vi "ACT_Loop.vi"() -> ()   [LabVIEW 2023, in "Grabber_ACT.lvlib"]
uses:
  Grabber_ACT.lvlib
  Cluster_CMD_ACT_Data.ctl
  Shared Code/TypeDefs/ENUM_Grabber_CMD_Mode Select.ctl
  Shared Code/TypeDefs/Cluster_Grabber_Config FX Values.ctl
  Shared Code/TypeDefs/Cluser_CAN Data.ctl
  Shared Code/TypeDefs/Cluster_Config Motor Output.ctl
  <vilib>/Rock Robotics/WPI/ThirdParty/Phoenix-LabVIEW/Motor Controller/Controls/CTRE_Phoenix_MotorControl_TalonFXInvertType.ctl
  <vilib>/Rock Robotics/WPI/ThirdParty/Phoenix-LabVIEW/Motor Controller/Controls/CTRE_Phoenix_MotorControl_NeutralMode.ctl
  Shared Code/TypeDefs/Cluster_FWD  REV Values.ctl
  Shared Code/TypeDefs/Cluser_FX Config_Current Limits.ctl
  Shared Code/TypeDefs/Cluster_Grabber HW Outputs.ctl
  Shared Code/TypeDefs/Cluster_FX Sensor Values.ctl
  Shared Code/TypeDefs/Cluster_FX CloseLoop Values.ctl
  Shared Code/TypeDefs/Cluster_FX Current Values.ctl
  Shared Code/TypeDefs/Cluster_Grabber_SW Outputs.ctl
  Shared Code/TypeDefs/Cluster_Grabber_Config SW Values.ctl
  ENUM_ACT_State.ctl
  <vilib>/Rock Robotics/WPI/MotorControl/WPI_MotorControlDeviceRef.ctl
  <vilib>/Rock Robotics/WPI/MotorControl/WPI_MotorControlType.ctl
  <vilib>/Rock Robotics/SystemInterfaces/DIO/FPGA_DIOPWMChannel.ctl
  <vilib>/Rock Robotics/WPI/PWM/WPI_PWMDeadband.ctl
  <vilib>/Rock Robotics/SystemInterfaces/DIO/FPGA_DIOChannel.ctl
  <vilib>/Rock Robotics/WPI/ThirdParty/Phoenix-LabVIEW/Motor Controller/Controls/CTRE_Phoenix_MotorControl_ControlMode.ctl
  ENUM_ACT_Action.ctl
  e7fa0f6b-fe57-4250-9995-b404d65a8362.vi
  4f1f8321-3dc8-4b28-8619-20673fc77ec2.vi
  6201c2b1-dcd8-4430-86f1-9b4ee56c7753.vi
  b5508d6c-c1cc-4273-80c5-2077d34e1483.vi
  36677ea0-a1a5-47a3-bc56-4475cb7c281e.vi
  5f725c2a-0ce1-4524-8967-e83b15fdce90.vi
  573e44c0-11f4-4bd9-ad56-904ec25dba75.vi
  e7494af9-f670-4352-9dfa-ae6ce50709ea.vi
  <vilib>/Utility/error.llb/Trim Whitespace.vi
  36677ea0-a1a5-47a3-bc56-4475cb7c281e.vi/958b2683-dd4b-41b7-8ed1-41c95f63cef0.vi
  36677ea0-a1a5-47a3-bc56-4475cb7c281e.vi/95f5fa9b-6175-4b34-88ee-cece92c38279.vi
  5f725c2a-0ce1-4524-8967-e83b15fdce90.vi/958b2683-dd4b-41b7-8ed1-41c95f63cef0.vi
  5f725c2a-0ce1-4524-8967-e83b15fdce90.vi/95f5fa9b-6175-4b34-88ee-cece92c38279.vi
  573e44c0-11f4-4bd9-ad56-904ec25dba75.vi/958b2683-dd4b-41b7-8ed1-41c95f63cef0.vi
  573e44c0-11f4-4bd9-ad56-904ec25dba75.vi/95f5fa9b-6175-4b34-88ee-cece92c38279.vi
  e7494af9-f670-4352-9dfa-ae6ce50709ea.vi/958b2683-dd4b-41b7-8ed1-41c95f63cef0.vi
  e7494af9-f670-4352-9dfa-ae6ce50709ea.vi/95f5fa9b-6175-4b34-88ee-cece92c38279.vi
  <vilib>/Utility/error.llb/Trim Whitespace One-Sided.vi
  36677ea0-a1a5-47a3-bc56-4475cb7c281e.vi/95f5fa9b-6175-4b34-88ee-cece92c38279.vi/1c6bd52c-bbca-4d4a-a290-93ea2703fded.vi
  36677ea0-a1a5-47a3-bc56-4475cb7c281e.vi/95f5fa9b-6175-4b34-88ee-cece92c38279.vi/47c2b0d5-b5fa-444e-9535-611565d375db.vi
  5f725c2a-0ce1-4524-8967-e83b15fdce90.vi/95f5fa9b-6175-4b34-88ee-cece92c38279.vi/1c6bd52c-bbca-4d4a-a290-93ea2703fded.vi
  5f725c2a-0ce1-4524-8967-e83b15fdce90.vi/95f5fa9b-6175-4b34-88ee-cece92c38279.vi/47c2b0d5-b5fa-444e-9535-611565d375db.vi
  573e44c0-11f4-4bd9-ad56-904ec25dba75.vi/95f5fa9b-6175-4b34-88ee-cece92c38279.vi/1c6bd52c-bbca-4d4a-a290-93ea2703fded.vi
  573e44c0-11f4-4bd9-ad56-904ec25dba75.vi/95f5fa9b-6175-4b34-88ee-cece92c38279.vi/47c2b0d5-b5fa-444e-9535-611565d375db.vi
  e7494af9-f670-4352-9dfa-ae6ce50709ea.vi/95f5fa9b-6175-4b34-88ee-cece92c38279.vi/1c6bd52c-bbca-4d4a-a290-93ea2703fded.vi
  e7494af9-f670-4352-9dfa-ae6ce50709ea.vi/95f5fa9b-6175-4b34-88ee-cece92c38279.vi/47c2b0d5-b5fa-444e-9535-611565d375db.vi
  RoboRIO Utilities/Global_STOP.vi
  Global_CMD_ACT_Data In.vi
  <vilib>/Utility/Data Type/Get Type Information.vi
  Shared Code/Utility/RWA/RWA/File/RWA_PC FIle Read String.vi
  Shared Code/Utility/RWA/RWA/Read Write Anything/RWA_File String.vi
  Shared Code/Utility/RWA/RWA/File/RWA_PC File Write String.vi
  Global_ACT_Data Out.vi
  <vilib>/Comparison/Equal/Equal Functor/Equal Functor.lvclass
panel:
  in  "Positon GO":bool
  in  "CMD Override":enum32{"None", "Intake", "Eject", "STOP"}(tab)
  out "Current Time":timestamp
  in  "SW Config":T1={"GrabberSW Ver"=230304152401, "Intake Speed"=0.4, "Eject Speed"=0.1, "Current Limit Velocity"=-12000, "Current Limit"=4.0, "Current Starting"=40.0, "Max Full Time(S)"=0.5}
  out "SW Output":T2
  out "Sensor Read time":dbl format="%.3g"
  out "HW Outputs":T3
  in  "Read Saved Config":bool
  in  "Update Config":bool
  in  "HW Config":T7 {"Output"."Min"."REV" format="%.2f"; "Output"."Min"."FWD" format="%.2f"; "Output"."Max"."REV" format="%.2f"; "Output"."Max"."FWD" format="%.2f"}
  out "CMD":T14
  out "Cycle Time (S)":dbl format="%.3g"
  # "Intake"
  # "Eject"
  # "STOP"
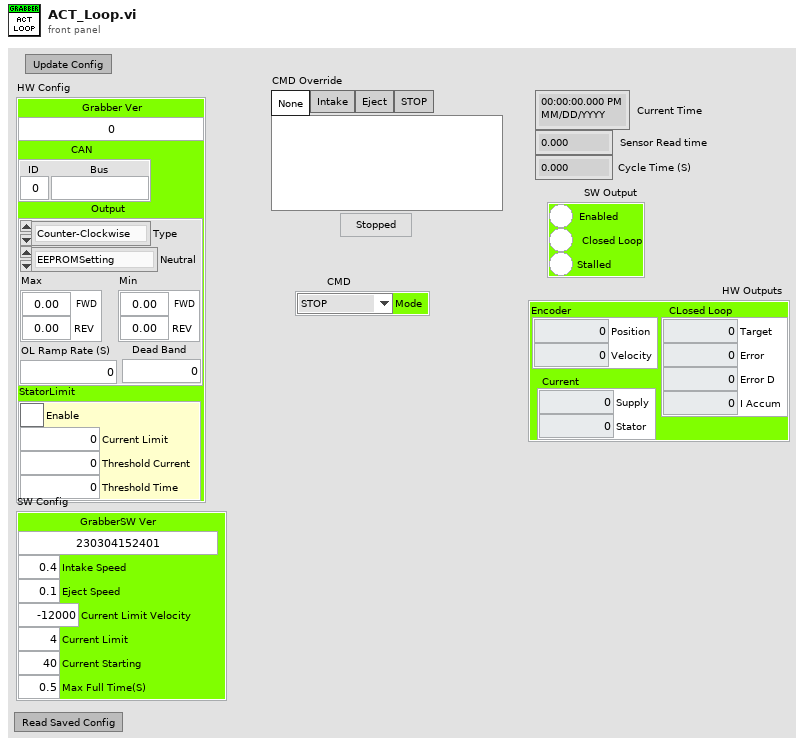
[diagram p1: front panel]
types:
  T1 = typedef "Cluster_Grabber_Config SW Values.ctl" = cluster{"GrabberSW Ver":u64, "Intake Speed":dbl, "Eject Speed":dbl, "Current Limit Velocity":i32, "Current Limit":dbl, "Current Starting":dbl, "Max Full Time(S)":dbl}
  T2 = typedef "Cluster_Grabber_SW Outputs.ctl" = cluster{"Enabled":bool, "Closed Loop":bool, "Stalled":bool}
  T3 = typedef "Cluster_Grabber HW Outputs.ctl" = cluster{"Encoder":T4, "CLosed Loop":T5, "Current":T6}
  T4 = typedef "Cluster_FX Sensor Values.ctl" = cluster{"Position":i32, "Velocity":i32}
  T5 = typedef "Cluster_FX CloseLoop Values.ctl" = cluster{"Target":dbl, "Error":i32, "Error D":dbl, "I Accum":dbl}
  T6 = typedef "Cluster_FX Current Values.ctl" = cluster{"Supply":dbl, "Stator":dbl}
  T7 = typedef "Cluster_Grabber_Config FX Values.ctl" = cluster{"Grabber Ver":u64, "CAN":T8, "Output":T9, "StatorLimit":T13}
  T8 = typedef "Cluser_CAN Data.ctl" = cluster{"ID":u8, "Bus":string}
  T9 = typedef "Cluster_Config Motor Output.ctl" = cluster{"Type":T10, "Neutral":T11, "Max":T12, "Min":T12, "OL Ramp Rate (S)":dbl, "Dead Band":dbl}
  T10 = typedef "CTRE_Phoenix_MotorControl_TalonFXInvertType.ctl" = enum16{"Counter-Clockwise", "Clockwise"}
  T11 = typedef "CTRE_Phoenix_MotorControl_NeutralMode.ctl" = enum8{"EEPROMSetting", "Override to Coast", "Override to Brake"}
  T12 = typedef "Cluster_FWD  REV Values.ctl" = cluster{"FWD":dbl, "REV":dbl}
  T13 = typedef "Cluser_FX Config_Current Limits.ctl" = cluster{"Enable":bool, "Current Limit":dbl, "Threshold Current":dbl, "Threshold Time":dbl}
  T14 = typedef "Grabber_ACT.lvlib/Cluster_CMD_ACT_Data.ctl" = cluster{"Mode":T15}
  T15 = typedef "ENUM_Grabber_CMD_Mode Select.ctl" = enum16{"STOP", "Intake", "Eject"}
  T16 = typedef "CTRE_Phoenix_MotorControl_ControlMode.ctl" = u16
  T17 = typedef "WPI_MotorControlDeviceRef.ctl" = cluster{"DeviceStatus":errorcluster, "Type":T18, "PWM":cluster{"PWM Channel":T19, "DeadBand":T20}, "CAN":cluster{"Device Number":u8, "SetOutput VI Ref":variant, "GetOutput VI Ref":variant, "Enable VI Ref":variant, "Disable VI Ref":variant, "Data":variant}, "Invert":bool, "DIO PWM":cluster{"PWM \"Enable\" Channel":T19, "DIOChannel":T21, "PWM Rate":dbl}}
  T18 = typedef "WPI_MotorControlType.ctl" = enum16{"PWM", "CAN", "DIO PWM"}
  T19 = typedef "FPGA_DIOPWMChannel.ctl" = enum8{"PWM 0", "PWM 1", "PWM 2", "PWM 3", "PWM 4", "PWM 5", "PWM 6", "PWM 7", "PWM 8", "PWM 9", "PWM MXP 0", "PWM MXP 1", "PWM MXP 2", "PWM MXP 3", "PWM MXP 4", "PWM MXP 5", "PWM MXP 6", "PWM MXP 7", "PWM MXP 8", "PWM MXP 9", "Invalid"}
  T20 = typedef "WPI_PWMDeadband.ctl" = cluster{"Name":string, "maxPositivePwm":i32, "minPositivePwm":i32, "centerPwm":i32, "maxNegativePwm":i32, "minNegativePwm":i32, "angularRange":u16}
  T21 = typedef "FPGA_DIOChannel.ctl" = enum8{"DIO 0", "DIO 1", "DIO 2", "DIO 3", "DIO 4", "DIO 5", "DIO 6", "DIO 7", "DIO 8", "DIO 9", "DIO MXP 0", "DIO MXP 1", "DIO MXP 2", "DIO MXP 3", "DIO MXP 4", "DIO MXP 5", "DIO MXP 6", "DIO MXP 7", "DIO MXP 8", "DIO MXP 9", "DIO MXP 10", "DIO MXP 11", "DIO MXP 12", "DIO MXP 13", "DIO MXP 14", "DIO MXP 15", "SPI Port CS1", "SPI Port CS2", "SPI Port CS3", "SPI Port MISO", "SPI Port MOSI", "Invalid"}
  T22 = typedef "Grabber_ACT.lvlib/ENUM_ACT_State.ctl" = enum16{"Startup", "Configuring", "Stopping", "Intaking Full", "Ejecting", "Shutdown", "Intake Limiting"}
  T23 = cluster{"Falcon Ref":T17, "State":T22, "Previous State":T22, "Current Time":timestamp, "Previous Time":timestamp, "Start Time":timestamp, "Target Time (ms)":u32, "Cycle Time(S)":dbl, "ACT Input":T14, "ACT Output DBL":dbl, "Team Files Folder":path, "HW Config":T7, "Update Display":bool, "Max # Of Config Tries":i32, "CAN Timeout":u32, "FX Mode":T16, "FX Set Value":dbl, "HW Outputs":T3, "SW Outputs":T2, "SW Config":T1}
  T24 = typedef "Grabber_ACT.lvlib/ENUM_ACT_Action.ctl" = enum16{"No Action", "Reset Time", "Reset All", "Config HW File Read", "Config HW File Save", "Config SW File Read", "Config SW File Save", "Config From FP", "Config HW Get", "Config HW Set", "Open HW Only", "Control FX Stop", "Control Eject", "Control Intake", "Set Current Limit"}
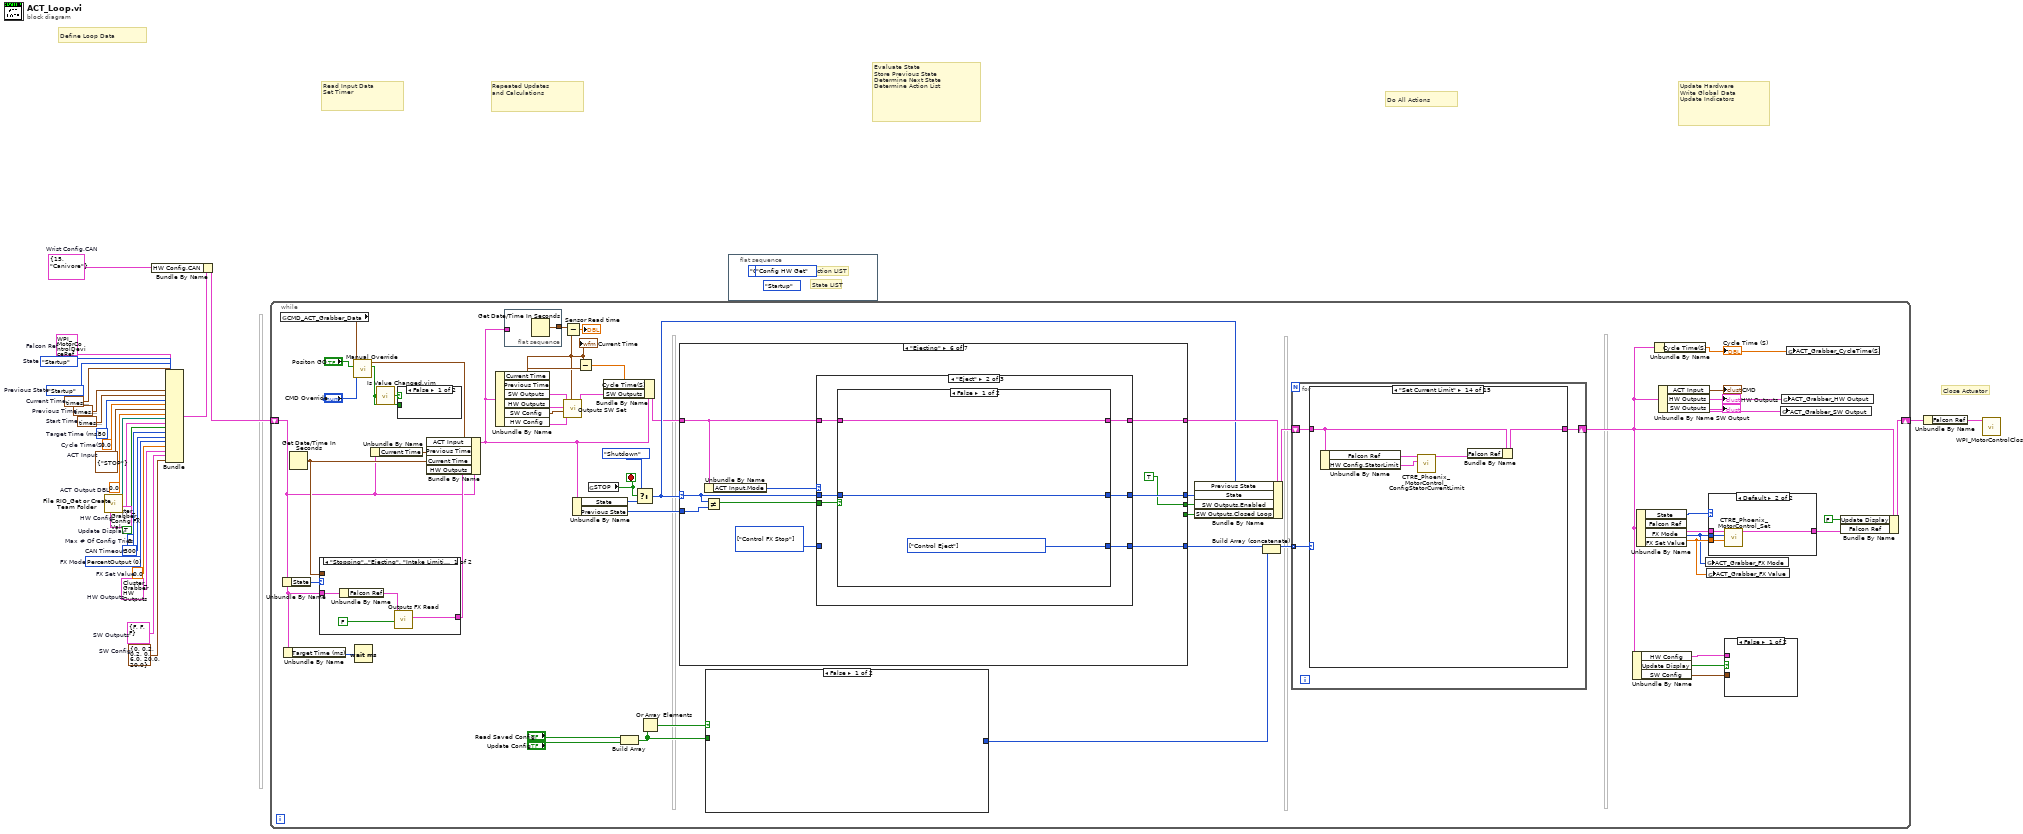
[diagram p0: block diagram]
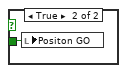
[diagram p2: hidden frame]
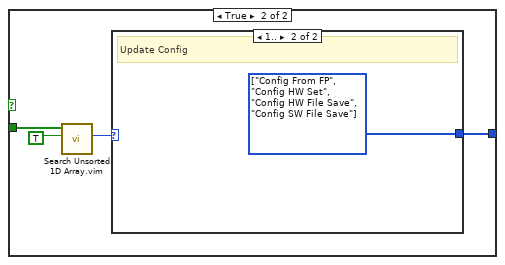
[diagram p4: hidden frame]
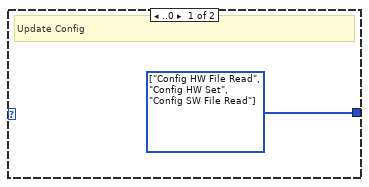
[diagram p5: hidden frame]
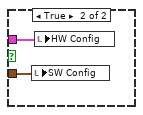
[diagram p7: hidden frame]
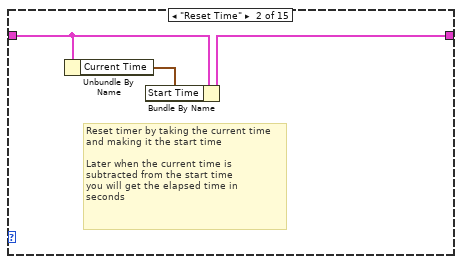
[diagram p9: hidden frame]
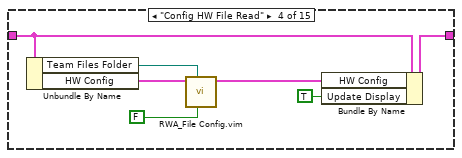
[diagram p11: hidden frame]
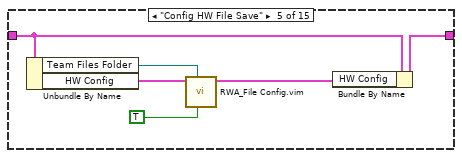
[diagram p12: hidden frame]
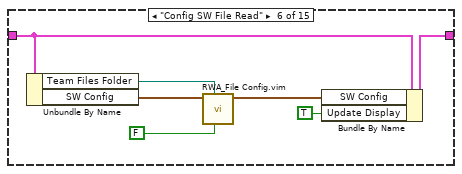
[diagram p13: hidden frame]
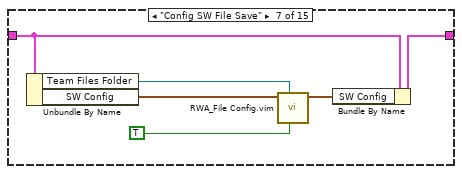
[diagram p14: hidden frame]
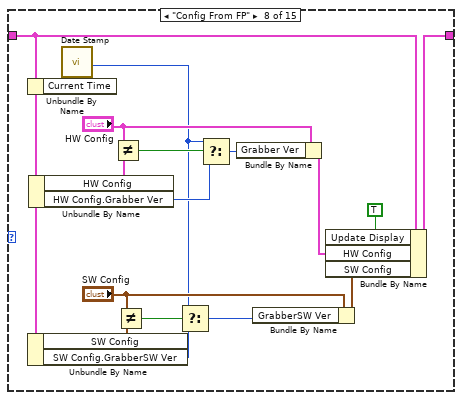
[diagram p15: hidden frame]
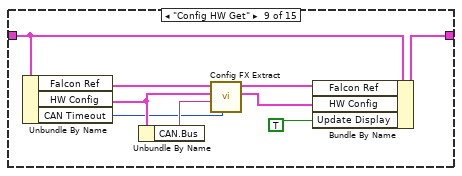
[diagram p16: hidden frame]
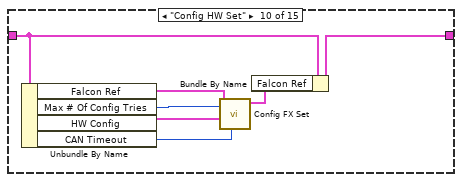
[diagram p17: hidden frame]
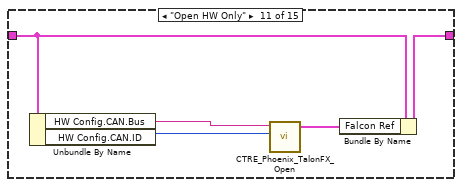
[diagram p18: hidden frame]
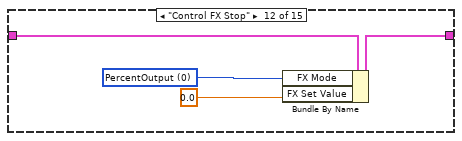
[diagram p19: hidden frame]
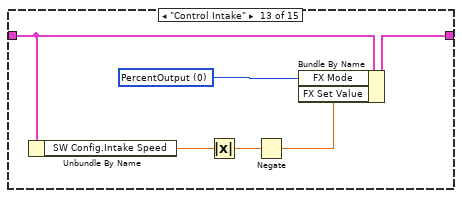
[diagram p20: hidden frame]
diagram:
  w1 = T1 {"GrabberSW Ver"=0, "Intake Speed"=0.2, "Eject Speed"=0.2, "Current Limit Velocity"=0, "Current Limit"=6.0, "Current Starting"=20.0, "Max Full Time(S)"=20.0}  # SW Config
  w2 = T2 {"Enabled"=FALSE, "Closed Loop"=FALSE, "Stalled"=FALSE}  # SW Outputs
  w3 = T3 {"Encoder"={"Position"=0, "Velocity"=0}, "CLosed Loop"={"Target"=0.0, "Error"=0, "Error D"=0.0, "I Accum"=0.0}, "Current"={"Supply"=0.0, "Stator"=0.0}}  # HW Outputs
  w5 = 0.0  # FX Set Value
  w6 = T16 0 items=["PercentOutput"=0, "Position"=1, "Velocity"=2, "Current"=3, "Follower"=5, "MotionProfile"=6, "MotionMagic"=7, "MotionProfileArc"=10, "Disabled"=15]  # FX Mode
  w7 = u32 300  # CAN Timeout
  w8 = 3  # Max # Of Config Tries
  w9 = TRUE  # Update Display
  w10 = T8 {"ID"=15, "Bus"="Canivore"}  # Wrist Config.CAN
  w11 = T7 {"Grabber Ver"=0, "CAN"={"ID"=0, "Bus"=""}, "Output"={"Type"=enum."Counter-Clockwise", "Neutral"=enum."EEPROMSetting", "Max"={"FWD"=0.0, "REV"=0.0}, "Min"={"FWD"=0.0, "REV"=0.0}, "OL Ramp Rate (S)"=0.0, "Dead Band"=0.0}, "StatorLimit"={"Enable"=FALSE, "Current Limit"=0.0, "Threshold Current"=0.0, "Threshold Time"=0.0}}  # HW Config
  w13 = T17 {"DeviceStatus"={"status"=FALSE, "code"=0, "source"=""}, "Type"=enum."PWM", "PWM"={"PWM Channel"=enum."PWM 1", "DeadBand"={"Name"="", "maxPositivePwm"=0, "minPositivePwm"=0, "centerPwm"=0, "maxNegativePwm"=0, "minNegativePwm"=0, "angularRange"=0}}, "CAN"={"Device Number"=0, "SetOutput VI Ref"=variant(enum8{"Percent VBus", "Current", "Speed", "Position", "Voltage"} enum."Percent VBus"), "GetOutput VI Ref"=variant(refnum<k1> refnum), "Enable VI Ref"=variant(dbl 12.0), "Disable VI Ref"=variant(enum8{"Percent VBus", "Speed", "Position", "Slave", "Unchanged / Invalid", "Voltage Compensation", "Current", "Motion Profile"} enum."Percent VBus"), "Data"=variant}, "Invert"=FALSE, "DIO PWM"={"PWM \"Enable\" Channel"=enum."Invalid", "DIOChannel"=enum."Invalid", "PWM Rate"=0.0}}  # Falcon Ref
  w17 = 0.0  # Cycle Time(S)
  w18 = ENUM_ACT_State."Startup"  # Previous State
  w19 = timestamp(0 s since 1904-01-01)  # Previous Time
  w20 = u32 50  # Target Time (ms)
  w21 = 0.0  # ACT Output DBL
  w22 = T14 {"Mode"=enum."STOP"}  # ACT Input
  w23 = timestamp(0 s since 1904-01-01)  # Start Time
  w24 = timestamp(0 s since 1904-01-01)  # Current Time
  w25 = ENUM_ACT_State."Startup"  # State
  # "Close Actuator"
  # "Define Loop Data"
  # "Repeated Updates\nand Calculations"
  # "Read Input Data\nSet Timer"
  # "Evaluate State\nStore Previous State\nDetermine Next State\nDetermine Action List"
  # "Do All Actions"
  # "Update Hardware\nWrite Global Data\nUpdate Indicators"
  n1 = call "File RIO_Get or Create Team Folder.vi"() -> ("Team Files Folder"=w12:path)  [unwired: 10 in, 1 out]
  n2 = Bundle("Falcon Ref"=w13, "State"=w25, "Previous State"=w18, "Current Time"=w24, "Previous Time"=w19, "Start Time"=w23, "Target Time (ms)"=w20, "Cycle Time(S)"=w17, "ACT Input"=w22, "ACT Output DBL"=w21, "Team Files Folder"=w12, "HW Config"=w11, "Update Display"=w9, "Max # Of Config Tries"=w8, "CAN Timeout"=w7, "FX Mode"=w6, "FX Set Value"=w5, "HW Outputs"=w3, "SW Outputs"=w2, "SW Config"=w1) -> (w15:T23)  [unwired: 1 in]
  n3 = Bundle By Name(cluster=w15, "HW Config.CAN"=w10) -> (w14:T23)
  n4 = while {
    shift-right: [w64] -> w16
    shift-left: w14 -> [w33]
    stop <- w78 stop-if-true
    n5 = global read "Global_CMD_ACT_Data In.vi" "CMD_ACT_Grabber_Data"() -> (w27:T14)
    n6 = Unbundle By Name(w33) -> ("State"=w54:T22)
    n7 = Unbundle By Name(w33) -> ("Target Time (ms)"=w75:u32)
    n8 = Get Date/Time In Seconds() -> (seconds since 1Jan1904=w50:timestamp)
    n9 = case shown="\"Stopping\"..\"Ejecting\", \"Intake Limiting\"" w54 {
      tunnel: w33 -> [w87 _]
      tunnel: w50 -> [_ _]
      tunnel: [w84 _] -> w34
      frame "Stopping".."Ejecting", "Intake Limiting" {
        n10 = Unbundle By Name(w87) -> ("Falcon Ref"=w86:T17)
        n11 = call "Outputs FX Read.vi"("Read Closed Loop"=FALSE, "Ref"=w86) -> ("Sensor Values Out"=w84:T3)  [unwired: 7 in, 2 out]
      }
      frame "Startup", "Configuring", "Shutdown" {
      }
    }
    n12 = call "Manual Override.vi"("Override"="CMD Override", "Position GO"="Positon GO", "Auto CMD"=w27) -> ("Position GO Out"=w31:bool, "OverRide Command Out"=w28:T14)  [unwired: 7 in]
    n13 = Wait (ms)(milliseconds to wait=w75) -> ()  [unwired: 1 out]
    n14 = Unbundle By Name(w33) -> ("Current Time"=w74:timestamp)
    n15 = call "Is Value Changed.vim"("value"=w31) -> ("changed or first call?"=w32:bool)
    n16 = case shown="False" w32 {
      tunnel: w31 -> [_ w82]
      frame False {
      }
      frame True {
        n17 = local write "Positon GO"(w82) -> ()
      }
    }
    n18 = Bundle By Name(cluster=w33, "ACT Input"=w28, "Previous Time"=w74, "Current Time"=w50, "HW Outputs"=w34) -> (w35:T23)
    n19 = Unbundle By Name(w35) -> ("Current Time"=w38:timestamp, "Previous Time"=w71:timestamp, "SW Outputs"=w41:T2, "HW Outputs"=w39:T3, "SW Config"=w26:T1, "HW Config"=w37:T7)
    "Current Time" <- w38
    n20 = flat-sequence {
      tunnel: [w83] -> w52
      tunnel: w35 -> [_]
      frame #0 {
        n21 = Get Date/Time In Seconds() -> (seconds since 1Jan1904=w83:timestamp)
      }
    }
    n22 = call "Outputs SW Set.vi"("Current Time"=w38, "Grabber Config"=w37, "SW Config"=w26, "Sensor Values"=w39, "SW Output"=w41) -> ("SW Output Out"=w40:T2)  [unwired: 6 in]
    n23 = Subtract(x=w52, y=w38) -> (x-y=→"Sensor Read time":dbl)
    n24 = Unbundle By Name(w35) -> ("State"=w76:T22, "Previous State"=w73:T22)
    n25 = Subtract(x=w38, y=w71) -> (x-y=w69:dbl)
    n26 = global read "Global_STOP.vi" "STOP"() -> (w78:bool)
    n27 = Bundle By Name(cluster=w35, "Cycle Time(S)"=w69, "SW Outputs"=w40) -> (w70:T23)
    n28 = Build Array("Read Saved Config", "Update Config") -> (w46:bool[])
    n29 = Select(t=ENUM_ACT_State."Shutdown" ("State"), s=w78, f=w76) -> (s? t:f=w72:T22)
    n30 = Or Array Elements(Boolean array=w46) -> (logical OR=w47:bool)
    n31 = case shown="\"Ejecting\"" w72 {
      selector: w72 -> [_ _ _ w237 w301 w316 _]
      tunnel: w70 -> [w195 w201 w225 w248 w302 w321 w348]
      tunnel: [w195 w204 w224 w249 w303 w322 w348] -> w80
      tunnel: [ENUM_ACT_State."Configuring" ("State") w203 w223 w251 w305 w324 ENUM_ACT_State."Shutdown" ("State")] -> w79
      tunnel: [w194 w202 w221 w247 w300 w319 w346] -> w68
      tunnel: w73 -> [_ _ _ w238 _ w317 _]
      tunnel: [_ _ TRUE TRUE TRUE TRUE _] -> w43
      tunnel: [_ _ _ FALSE FALSE _ _] -> w42
      frame "Startup" {
        w194 = T24[] [enum."Reset Time"] items=["No Action", "Reset Time", "Reset All", "Config HW File Read", "Config HW File Save", "Config SW File Read", "Config SW File Save", "Config From FP", "Config HW Get", "Config HW Set", "Open HW Only", "Control FX Stop", "Control Eject", "Control Intake", "Set Current Limit"] ("Actions")
      }
      frame "Configuring" {
        n32 = Unbundle By Name(w201) -> ("SW Config"=w199:T1)
        n33 = Unbundle By Name(w201) -> ("Team Files Folder"=w198:path, "HW Config"=w206:T7)
        n34 = call "Config_Build Name.vim"("Config First Name"=w206) -> ("Cfg file"=w208:string)  [unwired: 9 in, 1 out]
        n35 = call "Config_Build Name.vim"("Config First Name"=w199) -> ("Cfg file"=w200:string)  [unwired: 9 in, 1 out]
        n36 = Build Path(base path=w198, name or relative path=w200) -> (appended path=w197:path)
        n37 = Build Path(base path=w198, name or relative path=w208) -> (appended path=w207:path)
        n38 = call <vilib>:"Check if File or Folder Exists.vi"("path"=w197) -> ("file or folder exists?"=w196:bool)  [unwired: 8 in, 2 out]
        n39 = call <vilib>:"Check if File or Folder Exists.vi"("path"=w207) -> ("file or folder exists?"=w205:bool)  [unwired: 8 in, 2 out]
        n40 = case shown="True" w205 {
          tunnel: w201 -> [w211 w215]
          tunnel: [w211 w215] -> w204
          tunnel: [ENUM_ACT_State."Configuring" ("State") w214] -> w203
          tunnel: [w209 w213] -> w202
          tunnel: w196 -> [_ w212]
          frame False {
            w209 = T24[] [enum."Open HW Only", enum."Config HW Get", enum."Config HW File Save"] items=["No Action", "Reset Time", "Reset All", "Config HW File Read", "Config HW File Save", "Config SW File Read", "Config SW File Save", "Config From FP", "Config HW Get", "Config HW Set", "Open HW Only", "Control FX Stop", "Control Eject", "Control Intake", "Set Current Limit"] ("Actions")
            # "HW Config File Not Found"
          }
          frame True {
            # "HW Config File Found"
            n41 = case shown="False" w212 {
              tunnel: [ENUM_ACT_State."Stopping" ("State") ENUM_ACT_State."Stopping" ("State")] -> w214
              tunnel: [w216 w218] -> w213
              frame False {
                w216 = T24[] [enum."Config SW File Save"] items=["No Action", "Reset Time", "Reset All", "Config HW File Read", "Config HW File Save", "Config SW File Read", "Config SW File Save", "Config From FP", "Config HW Get", "Config HW Set", "Open HW Only", "Control FX Stop", "Control Eject", "Control Intake", "Set Current Limit"] ("Actions")
                # "SW Config File NOT Found"
              }
              frame True {
                w218 = T24[] [enum."Config HW File Read", enum."Config HW Set", enum."Config SW File Read", enum."Reset All", enum."Control FX Stop"] items=["No Action", "Reset Time", "Reset All", "Config HW File Read", "Config HW File Save", "Config SW File Read", "Config SW File Save", "Config From FP", "Config HW Get", "Config HW Set", "Open HW Only", "Control FX Stop", "Control Eject", "Control Intake", "Set Current Limit"] ("Actions")
                # "SW Config File Found"
              }
            }
          }
        }
      }
      frame "Stopping" {
        w222 = T24[] [enum."Control FX Stop"] items=["No Action", "Reset Time", "Reset All", "Config HW File Read", "Config HW File Save", "Config SW File Read", "Config SW File Save", "Config From FP", "Config HW Get", "Config HW Set", "Open HW Only", "Control FX Stop", "Control Eject", "Control Intake", "Set Current Limit"] ("Actions")
        n42 = Unbundle By Name(w225) -> ("ACT Input.Mode"=w226:T15)
        n43 = case shown="\"Intake\"" w226 {
          tunnel: w225 -> [w229 w232 w235]
          tunnel: [w229 w232 w235] -> w224
          tunnel: [ENUM_ACT_State."Stopping" ("State") ENUM_ACT_State."Intaking Full" ("State") ENUM_ACT_State."Ejecting" ("State")] -> w223
          tunnel: [w227 w230 w233] -> w221
          tunnel: w222 -> [w227 w230 w233]
          frame "STOP" {
          }
          frame "Intake" {
          }
          frame "Eject" {
          }
        }
      }
      frame "Intaking Full" {
        w246 = T24[] [enum."Control FX Stop"] items=["No Action", "Reset Time", "Reset All", "Config HW File Read", "Config HW File Save", "Config SW File Read", "Config SW File Save", "Config From FP", "Config HW Get", "Config HW Set", "Open HW Only", "Control FX Stop", "Control Eject", "Control Intake", "Set Current Limit"] ("Actions")
        n44 = Unbundle By Name(w248) -> ("Current Time"=w241:timestamp, "Start Time"=w240:timestamp, "SW Config.Max Full Time(S)"=w239:dbl, "SW Config.Current Limit Velocity"=w242:i32, "HW Outputs.Encoder.Velocity"=w243:i32, "ACT Input.Mode"=w250:T15)
        n45 = Not Equal?(x=w237, y=w238) -> (x != y?=w236:bool)
        n46 = case shown="\"Intake\"" w250 {
          tunnel: [ENUM_ACT_State."Stopping" ("State") ENUM_ACT_State."Ejecting" ("State") w262] -> w251
          tunnel: w248 -> [w254 w257 w264]
          tunnel: [w254 w257 w263] -> w249
          tunnel: w237 -> [_ _ _]
          tunnel: [w252 w255 w267] -> w247
          tunnel: w246 -> [w252 w255 _]
          tunnel: w243 -> [_ _ w266]
          tunnel: w242 -> [_ _ w265]
          tunnel: w241 -> [_ _ w261]
          tunnel: w240 -> [_ _ w260]
          tunnel: w239 -> [_ _ w259]
          tunnel: w236 -> [_ _ w258]
          frame "STOP" {
          }
          frame "Eject" {
          }
          frame "Intake" {
            n47 = case shown="False" w258 {
              tunnel: [w282 w296] -> w267
              tunnel: w266 -> [w281 _]
              tunnel: w265 -> [w280 _]
              tunnel: w264 -> [w279 w295]
              tunnel: [w278 w294] -> w263
              tunnel: [w277 ENUM_ACT_State."Intaking Full" ("State")] -> w262
              tunnel: w261 -> [w276 _]
              tunnel: w260 -> [w275 _]
              tunnel: w259 -> [w273 _]
              frame False {
                # "Not first call"
                n48 = Absolute Value(x=w280) -> (abs(x)=w269:i32)
                n49 = Subtract(x=w276, y=w275) -> (x-y=w274:dbl)
                n50 = Absolute Value(x=w281) -> (abs(x)=w268:i32)
                n51 = Greater Or Equal?(x=w268, y=w269) -> (x >= y?=w271:bool)
                n52 = Greater Or Equal?(x=w274, y=w273) -> (x >= y?=w272:bool)
                n53 = Or(x=w272, y=w271) -> (x .or. y?=w270:bool)
                n54 = case shown="True" w270 {
                  tunnel: [w287 w290] -> w282
                  tunnel: w279 -> [w284 w289]
                  tunnel: [w285 w289] -> w278
                  tunnel: [ENUM_ACT_State."Intake Limiting" ("State") ENUM_ACT_State."Intaking Full" ("State")] -> w277
                  frame True {
                    w287 = T24[] [enum."Set Current Limit", enum."Control Intake"] items=["No Action", "Reset Time", "Reset All", "Config HW File Read", "Config HW File Save", "Config SW File Read", "Config SW File Save", "Config From FP", "Config HW Get", "Config HW Set", "Open HW Only", "Control FX Stop", "Control Eject", "Control Intake", "Set Current Limit"] ("Actions")
                    # "Velocity target reached"
                    n55 = Unbundle By Name(w284) -> ("SW Config.Current Limit"=w283:dbl)
                    n56 = Bundle By Name(cluster=w284, "HW Config.StatorLimit.Current Limit"=w283) -> (w285:T23)
                  }
                  frame False {
                    w290 = T24[] [enum."Control Intake"] items=["No Action", "Reset Time", "Reset All", "Config HW File Read", "Config HW File Save", "Config SW File Read", "Config SW File Save", "Config From FP", "Config HW Get", "Config HW Set", "Open HW Only", "Control FX Stop", "Control Eject", "Control Intake", "Set Current Limit"] ("Actions")
                    # "Not at Velocity"
                  }
                }
              }
              frame True {
                w296 = T24[] [enum."Set Current Limit", enum."Control Intake"] items=["No Action", "Reset Time", "Reset All", "Config HW File Read", "Config HW File Save", "Config SW File Read", "Config SW File Save", "Config From FP", "Config HW Get", "Config HW Set", "Open HW Only", "Control FX Stop", "Control Eject", "Control Intake", "Set Current Limit"] ("Actions")
                # "First Call"
                n57 = Unbundle By Name(w295) -> ("Current Time"=w291:timestamp, "SW Config.Current Starting"=w292:dbl)
                n58 = Bundle By Name(cluster=w295, "Start Time"=w291, "HW Config.StatorLimit.Current Limit"=w292) -> (w294:T23)
              }
            }
          }
        }
      }
      frame "Intake Limiting" {
        w299 = T24[] [enum."Control FX Stop"] items=["No Action", "Reset Time", "Reset All", "Config HW File Read", "Config HW File Save", "Config SW File Read", "Config SW File Save", "Config From FP", "Config HW Get", "Config HW Set", "Open HW Only", "Control FX Stop", "Control Eject", "Control Intake", "Set Current Limit"] ("Actions")
        n59 = Unbundle By Name(w302) -> ("ACT Input.Mode"=w304:T15)
        n60 = case shown="\"STOP\"" w304 {
          tunnel: [ENUM_ACT_State."Stopping" ("State") ENUM_ACT_State."Ejecting" ("State") ENUM_ACT_State."Intake Limiting" ("State")] -> w305
          tunnel: w302 -> [w308 w311 w312]
          tunnel: [w308 w311 w312] -> w303
          tunnel: w301 -> [_ _ _]
          tunnel: [w306 w309 w314] -> w300
          tunnel: w299 -> [w306 w309 _]
          frame "STOP" {
          }
          frame "Eject" {
          }
          frame "Intake" {
            w314 = T24[] [enum."Control Intake"] items=["No Action", "Reset Time", "Reset All", "Config HW File Read", "Config HW File Save", "Config SW File Read", "Config SW File Save", "Config From FP", "Config HW Get", "Config HW Set", "Open HW Only", "Control FX Stop", "Control Eject", "Control Intake", "Set Current Limit"] ("Actions")
          }
        }
      }
      frame "Ejecting" {
        w320 = T24[] [enum."Control FX Stop"] items=["No Action", "Reset Time", "Reset All", "Config HW File Read", "Config HW File Save", "Config SW File Read", "Config SW File Save", "Config From FP", "Config HW Get", "Config HW Set", "Open HW Only", "Control FX Stop", "Control Eject", "Control Intake", "Set Current Limit"] ("Actions")
        n61 = Unbundle By Name(w321) -> ("ACT Input.Mode"=w323:T15)
        n62 = Not Equal?(x=w316, y=w317) -> (x != y?=w315:bool)
        n63 = case shown="\"Eject\"" w323 {
          tunnel: [ENUM_ACT_State."Stopping" ("State") w331 ENUM_ACT_State."Intaking Full" ("State")] -> w324
          tunnel: w321 -> [w327 w329 w345]
          tunnel: [w327 w328 w345] -> w322
          tunnel: w316 -> [_ w332 _]
          tunnel: [w325 w333 w343] -> w319
          tunnel: w320 -> [w325 _ w343]
          tunnel: w315 -> [_ w330 _]
          frame "STOP" {
          }
          frame "Eject" {
            n64 = case shown="False" w330 {
              tunnel: [w334 w342] -> w333
              tunnel: w332 -> [w335 w341]
              tunnel: [w335 w341] -> w331
              tunnel: w329 -> [w336 w340]
              tunnel: [w336 w339] -> w328
              frame False {
                w334 = T24[] [enum."Control Eject"] items=["No Action", "Reset Time", "Reset All", "Config HW File Read", "Config HW File Save", "Config SW File Read", "Config SW File Save", "Config From FP", "Config HW Get", "Config HW Set", "Open HW Only", "Control FX Stop", "Control Eject", "Control Intake", "Set Current Limit"] ("Actions")
              }
              frame True {
                w342 = T24[] [enum."Set Current Limit", enum."Control Eject"] items=["No Action", "Reset Time", "Reset All", "Config HW File Read", "Config HW File Save", "Config SW File Read", "Config SW File Save", "Config From FP", "Config HW Get", "Config HW Set", "Open HW Only", "Control FX Stop", "Control Eject", "Control Intake", "Set Current Limit"] ("Actions")
                # "First Call"
                n65 = Unbundle By Name(w340) -> ("Current Time"=w337:timestamp, "SW Config.Current Starting"=w338:dbl)
                n66 = Bundle By Name(cluster=w340, "Start Time"=w337, "HW Config.StatorLimit.Current Limit"=w338) -> (w339:T23)
              }
            }
          }
          frame "Intake" {
          }
        }
      }
      frame "Shutdown" {
        w346 = T24[] [enum."Reset All"] items=["No Action", "Reset Time", "Reset All", "Config HW File Read", "Config HW File Save", "Config SW File Read", "Config SW File Save", "Config From FP", "Config HW Get", "Config HW Set", "Open HW Only", "Control FX Stop", "Control Eject", "Control Intake", "Set Current Limit"] ("Actions")
      }
    }
    n67 = case shown="False" w47 {
      tunnel: w46 -> [_ w90]
      tunnel: [_ w88] -> w45
      frame False {
      }
      frame True {
        n68 = call "Search Unsorted 1D Array.vim"("element"=TRUE, "unsorted 1D array"=w90) -> ("index of element"=w89:i32)  [unwired: 9 in]
        n69 = case shown="1.." w89 {
          tunnel: [w92 w93] -> w88
          frame ..0 {
            w92 = T24[] [enum."Config HW File Read", enum."Config HW Set", enum."Config SW File Read"] items=["No Action", "Reset Time", "Reset All", "Config HW File Read", "Config HW File Save", "Config SW File Read", "Config SW File Save", "Config From FP", "Config HW Get", "Config HW Set", "Open HW Only", "Control FX Stop", "Control Eject", "Control Intake", "Set Current Limit"] ("Actions")
            # "Update Config"
          }
          frame 1.. {
            w93 = T24[] [enum."Config From FP", enum."Config HW Set", enum."Config HW File Save", enum."Config SW File Save"] items=["No Action", "Reset Time", "Reset All", "Config HW File Read", "Config HW File Save", "Config SW File Read", "Config SW File Save", "Config From FP", "Config HW Get", "Config HW Set", "Open HW Only", "Control FX Stop", "Control Eject", "Control Intake", "Set Current Limit"] ("Actions")
            # "Update Config"
          }
        }
      }
    }
    n70 = Bundle By Name(cluster=w80, "Previous State"=w72, "State"=w79, "SW Outputs.Enabled"=w43, "SW Outputs.Closed Loop"=w42) -> (w81:T23)
    n71 = Build Array (concatenate)(w68, w45) -> (w62:T24[])
    n72 = for {
      tunnel: w62 -> [w103] mode=indexing
      shift-right: [w102] -> w61
      shift-left: w81 -> [w101]
      n73 = case shown="\"Set Current Limit\"" w103 {
        tunnel: w101 -> [w104 w107 w108 w114 w120 w127 w133 w141 w157 w165 w169 w175 w180 w187 w190]
        tunnel: [w104 w106 w108 w115 w121 w128 w134 w151 w158 w166 w170 w176 w182 w186 w192] -> w102
        frame "No Action" {
        }
        frame "Reset Time" {
          # "Reset timer by taking the current time\nand making it the start time\n\nLater when the current time is \nsubtracted from the start time\nyou will get the elapsed time in \nseconds"
          n74 = Unbundle By Name(w107) -> ("Current Time"=w105:timestamp)
          n75 = Bundle By Name(cluster=w107, "Start Time"=w105) -> (w106:T23)
        }
        frame "Reset All" {
        }
        frame "Config HW File Read" {
          n76 = Unbundle By Name(w114) -> ("Team Files Folder"=w111:path, "HW Config"=w113:T7)
          n77 = call "RWA_File Config.vim"("Read(f) Save(t)"=FALSE ("Read(f) Write(t)"), "Target Folder Folder"=w111, "Any Config"=w113) -> ("Any Config Out"=w112:T7)  [unwired: 4 in, 4 out]
          n78 = Bundle By Name(cluster=w114, "HW Config"=w112, "Update Display"=TRUE) -> (w115:T23)
        }
        frame "Config HW File Save" {
          n79 = Unbundle By Name(w120) -> ("Team Files Folder"=w117:path, "HW Config"=w119:T7)
          n80 = call "RWA_File Config.vim"("Read(f) Save(t)"=TRUE ("Read(f) Write(t)"), "Target Folder Folder"=w117, "Any Config"=w119) -> ("Any Config Out"=w118:T7)  [unwired: 4 in, 4 out]
          n81 = Bundle By Name(cluster=w120, "HW Config"=w118) -> (w121:T23)
        }
        frame "Config SW File Read" {
          n82 = Unbundle By Name(w127) -> ("Team Files Folder"=w124:path, "SW Config"=w126:T1)
          n83 = call "RWA_File Config.vim"("Read(f) Save(t)"=FALSE ("Read(f) Write(t)"), "Target Folder Folder"=w124, "Any Config"=w126) -> ("Any Config Out"=w125:T1)  [unwired: 4 in, 4 out]
          n84 = Bundle By Name(cluster=w127, "SW Config"=w125, "Update Display"=TRUE) -> (w128:T23)
        }
        frame "Config SW File Save" {
          n85 = Unbundle By Name(w133) -> ("Team Files Folder"=w130:path, "SW Config"=w132:T1)
          n86 = call "RWA_File Config.vim"("Read(f) Save(t)"=TRUE ("Read(f) Write(t)"), "Target Folder Folder"=w130, "Any Config"=w132) -> ("Any Config Out"=w131:T1)  [unwired: 4 in, 4 out]
          n87 = Bundle By Name(cluster=w133, "SW Config"=w131) -> (w134:T23)
        }
        frame "Config From FP" {
          n88 = Unbundle By Name(w141) -> ("Current Time"=w150:timestamp)
          n89 = Unbundle By Name(w141) -> ("SW Config"=w143:T1, "SW Config.GrabberSW Ver"=w145:u64)
          n90 = Unbundle By Name(w141) -> ("HW Config"=w140:T7, "HW Config.Grabber Ver"=w137:u64)
          n91 = call "Date Stamp.vi"("Time"=w150) -> ("U64 Out"=w136:u64)  [unwired: 5 in, 1 out]
          n92 = Not Equal?(x="HW Config", y=w140) -> (x != y?=w138:bool)
          n93 = Not Equal?(x=w143, y="SW Config") -> (x != y?=w146:bool)
          n94 = Select(t=w136, s=w146, f=w145) -> (s? t:f=w144:u64)
          n95 = Select(t=w136, s=w138, f=w137) -> (s? t:f=w135:u64)
          n96 = Bundle By Name(cluster="HW Config", "Grabber Ver"=w135) -> (w149:T7)
          n97 = Bundle By Name(cluster="SW Config", "GrabberSW Ver"=w144) -> (w148:T1)
          n98 = Bundle By Name(cluster=w141, "Update Display"=TRUE, "HW Config"=w149, "SW Config"=w148) -> (w151:T23)
        }
        frame "Config HW Get" {
          n99 = Unbundle By Name(w157) -> ("Falcon Ref"=w160:T17, "HW Config"=w154:T7, "CAN Timeout"=w152:u32)
          n100 = Unbundle By Name(w154) -> ("CAN.Bus"=w159:string)
          n101 = call "Config FX Extract.vi"("Send Cmd Timout(ms)"=w152, "CAN.Bus"=w159, "Config"=w154, "PhoenixMotorControlDevRef"=w160) -> ("Config Data Out"=w153:T7, "Module Azimuth Ref Out"=w156:T17)  [unwired: 5 in, 1 out]
          n102 = Bundle By Name(cluster=w157, "Falcon Ref"=w156, "HW Config"=w153, "Update Display"=TRUE) -> (w158:T23)
        }
        frame "Config HW Set" {
          n103 = Unbundle By Name(w165) -> ("Falcon Ref"=w167:T17, "Max # Of Config Tries"=w162:i32, "HW Config"=w161:T7, "CAN Timeout"=w163:u32)
          n104 = call "Config FX Set.vi"("Max # Of Tries"=w162, "Send Cmd Timout(ms)"=w163, "Grabber Config"=w161, "PhoenixMotorControlDevRef"=w167) -> ("PhoenixMotorControlDevRef Out Out"=w164:T17)  [unwired: 6 in, 1 out]
          n105 = Bundle By Name(cluster=w165, "Falcon Ref"=w164) -> (w166:T23)
        }
        frame "Open HW Only" {
          n106 = Unbundle By Name(w169) -> ("HW Config.CAN.Bus"=w168:string, "HW Config.CAN.ID"=w172:u8)
          n107 = call <vilib>:"CTRE_Phoenix_TalonFX_Open.vi"("Device Number"=w172, "CAN Bus"=w168) -> ("PhoenixMotorControlDevRef"=w171:T17)  [unwired: 8 in, 1 out]
          n108 = Bundle By Name(cluster=w169, "Falcon Ref"=w171) -> (w170:T23)
        }
        frame "Control FX Stop" {
          w174 = T16 0 items=["PercentOutput"=0, "Position"=1, "Velocity"=2, "Current"=3, "Follower"=5, "MotionProfile"=6, "MotionMagic"=7, "MotionProfileArc"=10, "Disabled"=15] ("FX Mode")
          n109 = Bundle By Name(cluster=w175, "FX Mode"=w174, "FX Set Value"=0.0) -> (w176:T23)
        }
        frame "Control Intake" {
          w181 = T16 0 items=["PercentOutput"=0, "Position"=1, "Velocity"=2, "Current"=3, "Follower"=5, "MotionProfile"=6, "MotionMagic"=7, "MotionProfileArc"=10, "Disabled"=15] ("FX Mode")
          n110 = Unbundle By Name(w180) -> ("SW Config.Intake Speed"=w179:dbl)
          n111 = Absolute Value(x=w179) -> (abs(x)=w178:dbl)
          n112 = Negate(x=w178) -> (-x=w177:dbl)
          n113 = Bundle By Name(cluster=w180, "FX Mode"=w181, "FX Set Value"=w177) -> (w182:T23)
        }
        frame "Set Current Limit" {
          n114 = Unbundle By Name(w187) -> ("Falcon Ref"=w185:T17, "HW Config.StatorLimit"=w183:T13)
          n115 = call <vilib>:"CTRE_Phoenix_MotorControl_ConfigStatorCurrentLimit.vi"("Stator Current Limit Configuration"=w183, "PhoenixMotorControlDevRef"=w185) -> ("PhoenixMotorControlDevRef"=w184:T17)  [unwired: 8 in, 1 out]
          n116 = Bundle By Name(cluster=w187, "Falcon Ref"=w184) -> (w186:T23)
        }
        frame "Control Eject" {
          w191 = T16 0 items=["PercentOutput"=0, "Position"=1, "Velocity"=2, "Current"=3, "Follower"=5, "MotionProfile"=6, "MotionMagic"=7, "MotionProfileArc"=10, "Disabled"=15] ("FX Mode")
          n117 = Unbundle By Name(w190) -> ("SW Config.Eject Speed"=w189:dbl)
          n118 = Absolute Value(x=w189) -> (abs(x)=w188:dbl)
          n119 = Bundle By Name(cluster=w190, "FX Mode"=w191, "FX Set Value"=w188) -> (w192:T23)
        }
      }
    }
    n120 = Unbundle By Name(w61) -> ("HW Config"=w58:T7, "Update Display"=w59:bool, "SW Config"=w36:T1)
    n121 = Unbundle By Name(w61) -> ("State"=w55:T22, "Falcon Ref"=w66:T17, "FX Mode"=w56:T16, "FX Set Value"=w57:dbl)
    n122 = Unbundle By Name(w61) -> ("Cycle Time(S)"=w63:dbl)
    "Cycle Time (S)" <- w63
    n123 = Unbundle By Name(w61) -> ("ACT Input"=→"CMD":T14, "HW Outputs"=w53:T3, "SW Outputs"=w44:T2)
    "HW Outputs" <- w53
    "SW Output" <- w44
    n124 = global write "Global_ACT_Data Out.vi" "ACT_Grabber_FX Mode"(w56) -> ()
    n125 = global write "Global_ACT_Data Out.vi" "ACT_Grabber_FX Value"(w57) -> ()
    n126 = case shown="Default" w55 {
      tunnel: w66 -> [w94 w98]
      tunnel: [w94 w97] -> w65
      tunnel: w57 -> [_ w96]
      tunnel: w56 -> [_ w95]
      frame "Startup", "Configuring" {
      }
      frame Default {
        n127 = call <vilib>:"CTRE_Phoenix_MotorControl_Set.vi"("Output"=w96, "Control Mode"=w95, "PhoenixMotorControlDevRef"=w98) -> ("PhoenixMotorControlDevRef"=w97:T17)  [unwired: 7 in, 1 out]
      }
    }
    n128 = case shown="False" w59 {
      tunnel: w58 -> [_ w100]
      tunnel: w36 -> [_ w99]
      frame False {
      }
      frame True {
        n129 = local write "SW Config"(w99) -> ()
        n130 = local write "HW Config"(w100) -> ()
      }
    }
    n131 = global write "Global_ACT_Data Out.vi" "ACT_Grabber_SW Output"(w44) -> ()
    n132 = global write "Global_ACT_Data Out.vi" "ACT_Grabber_HW Output"(w53) -> ()
    n133 = global write "Global_ACT_Data Out.vi" "ACT_Grabber_CycleTime(S)"(w63) -> ()
    n134 = Bundle By Name(cluster=w61, "Update Display"=FALSE, "Falcon Ref"=w65) -> (w64:T23)
  }
  n135 = flat-sequence {
    frame #0 {
      (unwired) ENUM_ACT_Action."Open HW Only" ("Action")
      (unwired) ENUM_ACT_State."Startup" ("State")
      (unwired) ENUM_ACT_Action."Config HW Get" ("Action")
      # "State LIST"
      # "Action LIST"
    }
  }
  n136 = Unbundle By Name(w16) -> ("Falcon Ref"=w4:T17)
  n137 = call <vilib>:"WPI_MotorControlClose.vi"("MotorControlDevRef"=w4) -> ()  [unwired: 10 in, 1 out]
